vi "subIsDelimiterNameContainer.vi"(11 "delimited name":string) -> (1 "Is a container?":bool, 2 "item name":string, 3 "container name[]":string[](array[string]))   [LabVIEW 2020, in "LabVIEWItem.lvlib" / "CLabVIEWItem.lvclass"]
uses:
  CLabVIEWItem.lvclass
  <vilib>/regexp/Match Regular Expression.xnode
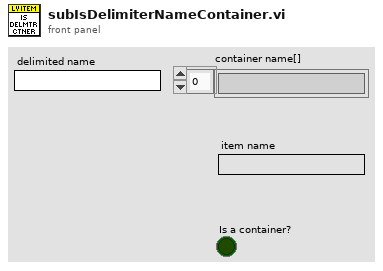
[diagram p1: front panel]
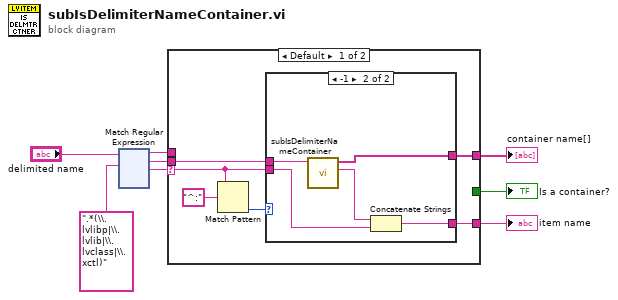
[diagram p0: block diagram]
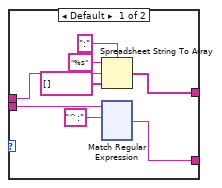
[diagram p2: hidden frame]
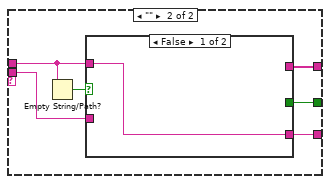
[diagram p3: hidden frame]
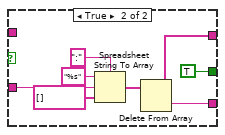
[diagram p4: hidden frame]
diagram:
  n1 = xnode "Match Regular Expression"("input string"="delimited name", "regular expression"=".*(\\.lvlibp|\\.lvlib|\\.lvclass|\\.xctl)") -> ("before match"=w2:string, "whole match"=w3:string, "after match"=w4:string)  [unwired: 4 in, 2 out]
  n2 = case shown="Default" w4 {
    selector: w4 -> [w12 _]
    tunnel: [_ w147] -> w8
    tunnel: w3 -> [w11 w146]
    tunnel: [w9 w145] -> w7
    tunnel: [w10 w144] -> w5
    tunnel: w2 -> [_ w142]
    frame Default {
      n3 = Match Pattern(string=w12, regular expression="^:") -> (offset past match=w13:i32)  [unwired: 1 in, 3 out]
      n4 = case shown="-1" w13 {
        tunnel: w12 -> [w17 w139]
        tunnel: w11 -> [w18 w141]
        tunnel: [w16 w137] -> w10
        tunnel: [w15 w138] -> w9
        frame Default {
          n5 = Spreadsheet String To Array(delimiter (Tab)=":", format string="%s", spreadsheet string=w18, array type (2D Dbl)=string[] []) -> (array=w16:string[])
          n6 = xnode "Match Regular Expression"("input string"=w17, "regular expression"="^:") -> ("after match"=w15:string)  [unwired: 4 in, 4 out]
        }
        frame -1 {
          n7 = call "subIsDelimiterNameContainer.vi"("delimited name"=w141) -> ("item name"=w140:string, "container name[]"=w137:string[])  [unwired: 8 in, 1 out]
          n8 = Concatenate Strings(w140, w139) -> (w138:string)
        }
      }
    }
    frame "" {
      n9 = Empty String/Path?(string/path=w142) -> (empty?=w143:bool)
      n10 = case shown="False" w143 {
        tunnel: [_ TRUE] -> w147
        tunnel: w146 -> [_ w152]
        tunnel: [w148 w150] -> w145
        tunnel: [_ w149] -> w144
        tunnel: w142 -> [w148 _]
        frame False {
        }
        frame True {
          n11 = Spreadsheet String To Array(delimiter (Tab)=":", format string="%s", spreadsheet string=w152, array type (2D Dbl)=string[] []) -> (array=w151:string[])
          n12 = Delete From Array(array=w151) -> (deleted portion=w150:string, array with subset deleted=w149:string[])  [unwired: 2 in]
        }
      }
    }
  }
  "Is a container?" <- w8
  "item name" <- w7
  "container name[]" <- w5
